vi "Compute angle.vi"(8 "error in (no error)":errorcluster, 11 "AOTF in":refnum<class "AOTF.lvclass">) -> (0 "error out":errorcluster, 2 "Angle":sgl, 3 "AOTF out":refnum<class "AOTF.lvclass">)   [LabVIEW 2012, in "AOTF.lvclass"]
uses:
  AOTF.lvclass
  Controls/Illumination arm.ctl
  AOTF.lvclass/AOTF.ctl
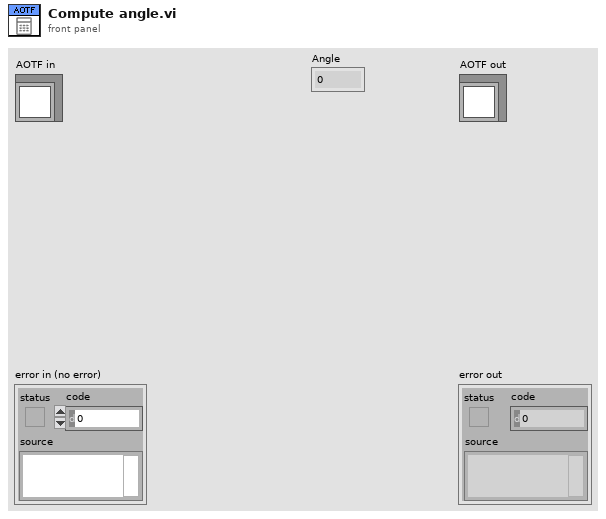
[diagram p1: front panel]
types:
  T1 = typedef "AOTF.lvclass/Illumination arm.ctl" = enum16{"Florence", "Prato"}
  T2 = typedef "AOTF.lvclass/laser line ring.ctl" = u8
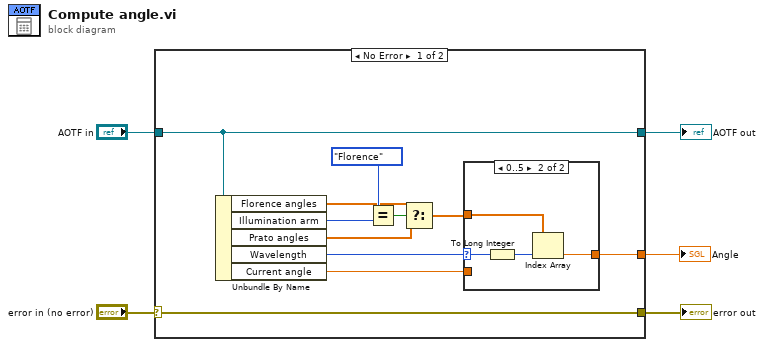
[diagram p0: block diagram]
diagram:
  n1 = case shown="No Error" "error in (no error)" {
    selector: "error in (no error)" -> [w16 w23]
    tunnel: [w16 w23] -> w4
    tunnel: [w15 w22] -> w2
    tunnel: "AOTF in" -> [w15 w22]
    tunnel: [w12 _] -> w1
    frame No Error {
      n2 = Unbundle By Name(w15) -> ("Florence angles"=w9:sgl[], "Illumination arm"=w10:T1, "Prato angles"=w8:sgl[], "Wavelength"=w11:T2, "Current angle"=w6:sgl)
      n3 = Equal?(x=Illumination_arm."Florence", y=w10) -> (x = y?=w14:bool)
      n4 = Select(t=w9, s=w14, f=w8) -> (s? t:f=w7:sgl[])
      n5 = case shown="0..5" w11 {
        selector: w11 -> [_ w19]
        tunnel: w7 -> [_ w21]
        tunnel: [w17 w20] -> w12
        tunnel: w6 -> [w17 _]
        frame 10, Default {
        }
        frame 0..5 {
          n6 = To Long Integer(number=w19) -> (32bit integer=w18:i32)
          n7 = Index Array(array=w21, index=w18) -> (element=w20:sgl)
        }
      }
    }
    frame Error {
    }
  }
  "error out" <- w4
  "AOTF out" <- w2
  "Angle" <- w1
